vi "genIOLInsertion.vi"(11 "Arm ID Ind":i32) -> (0 "zVisTraj":dbl[](array[numeric]) format="%_6g", 1 "yVisTraj":dbl[](array[numeric]) format="%_6g", 2 "xVisTraj":dbl[](array[numeric]) format="%_6g")   [LabVIEW 2016]
uses:
  <vilib>/Analysis/NI_AALBase.lvlib
  <vilib>/Analysis/1siggen.llb/Ramp Pattern by Samples.vi
  <vilib>/gmath/NI_Gmath.lvlib
panel:
  in  "Total Time":dbl=60.0
  in  "Tip out Posit":dbl[](array[numeric])=[0.0, 0.0, 0.0] caption="Position [mm]" format="%#.3f"
  in  "Cycle Time [sec]":dbl[](array[numeric])=[60.0, 90.0, 120.0]
  in  "Sampling Rate [Hz]":i32=1000
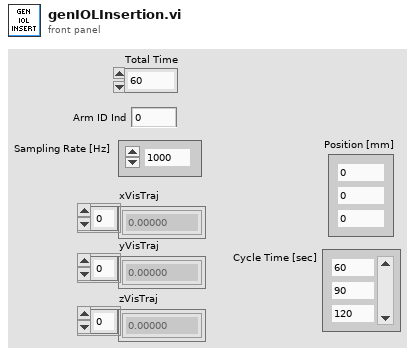
[diagram p1: front panel]
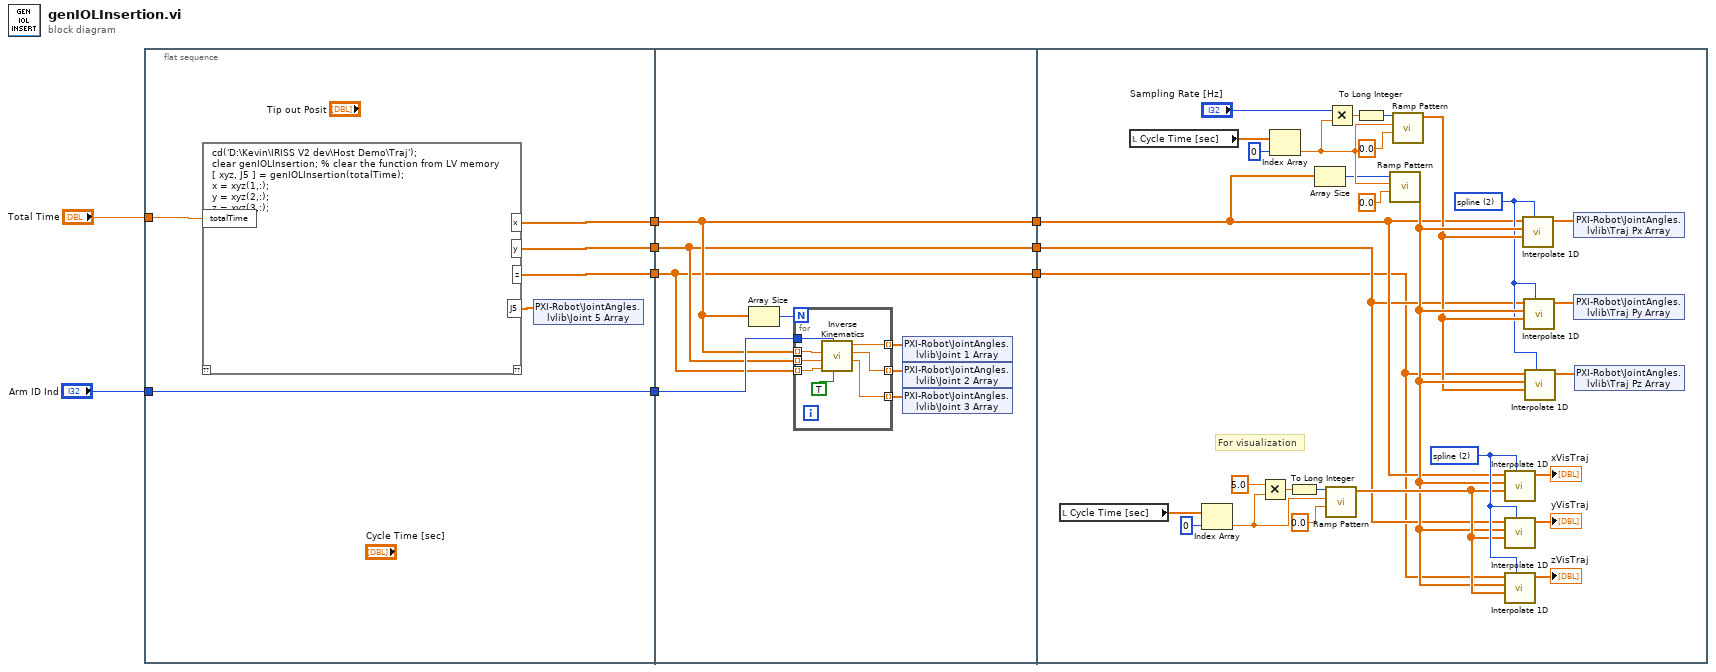
[diagram p0: block diagram]
diagram:
  n1 = flat-sequence {
    tunnel: "Arm ID Ind" -> [w14]
    tunnel: [w14] -> w8
    tunnel: [w13] -> w4
    tunnel: [w12] -> w3
    tunnel: [w11] -> w2
    tunnel: "Total Time" -> [w10]
    tunnel: w8 -> [w23]
    tunnel: [w18] -> w7
    tunnel: [w17] -> w6
    tunnel: [w16] -> w5
    tunnel: w4 -> [w18]
    tunnel: w3 -> [w17]
    tunnel: w2 -> [w16]
    tunnel: w7 -> [w34]
    tunnel: w6 -> [w33]
    tunnel: w5 -> [w32]
    frame #0 {
      n2 = script code="cd('D:\\Kevin\\IRISS V2 dev\\Host Demo\\Traj');\nclear genIOLInsertion; % clear the function from LV memory\n[ xyz, J5 ] = genIOLInsertion(totalTime);\nx = xyz(1,:);\ny = xyz(2,:);\nz = xyz(3,:);"("totalTime"=w10) -> ("x"=w13:dbl[], "y"=w12:dbl[], "z"=w11:dbl[], "J5"=w15:dbl[])  [unwired: 1 in, 1 out]
      n3 = shared-variable "PXI-Robot\\JointAngles.lvlib\\Joint 5 Array"(w15) -> ()  [unwired: 1 in, 1 out]
    }
    frame #1 {
      n4 = Array Size(array=w18) -> (size(s)=w22:i32)
      n5 = for {
        N: w22 -> [_]
        tunnel: w23 -> [w27]
        tunnel: w18 -> [w31] mode=indexing
        tunnel: w17 -> [w30] mode=indexing
        tunnel: w16 -> [w29] mode=indexing
        tunnel: [w26] -> w21 mode=indexing
        tunnel: [w25] -> w20 mode=indexing
        tunnel: [w24] -> w19 mode=indexing
        n6 = call "Inverse Kinematics.vi"(6:TRUE ("isToolTipInsideEye"), "armID"=w27, "z"=w29, "y"=w30, "x"=w31) -> ("j3"=w24:dbl, "j2"=w25:dbl, "j1"=w26:dbl)  [unwired: 3 in, 1 out]
      }
      n7 = shared-variable "PXI-Robot\\JointAngles.lvlib\\Joint 1 Array"(w21) -> ()  [unwired: 1 in, 1 out]
      n8 = shared-variable "PXI-Robot\\JointAngles.lvlib\\Joint 2 Array"(w20) -> ()  [unwired: 1 in, 1 out]
      n9 = shared-variable "PXI-Robot\\JointAngles.lvlib\\Joint 3 Array"(w19) -> ()  [unwired: 1 in, 1 out]
    }
    frame #2 {
      w49 = 2 items=["nearest", "linear", "spline", "cubic Hermite", "Lagrange"] ("method")
      w35 = 2 items=["nearest", "linear", "spline", "cubic Hermite", "Lagrange"] ("method")
      # "For visualization"
      n10 = local read "Cycle Time [sec]"() -> (w43:dbl[])
      n11 = local read "Cycle Time [sec]"() -> (w61:dbl[])
      n12 = Index Array(array=w43, index=0) -> (element=w44:dbl)
      n13 = Multiply(x=5.0, y=w44) -> (x*y=w46:dbl)
      n14 = Index Array(array=w61, index=0) -> (element=w54:dbl)
      n15 = To Long Integer(number=w46) -> (32bit integer=w47:i32)
      n16 = Array Size(array=w34) -> (size(s)=w53:i32)
      n17 = call-poly <vilib>:"Ramp Pattern.vi"("start"=0.0, "end"=w44, "samples"=w47) -> ("Ramp Pattern"=w41:dbl[])  [unwired: 7 in, 1 out]
      n18 = Multiply(x="Sampling Rate [Hz]", y=w54) -> (x*y=w57:dbl)
      n19 = To Long Integer(number=w57) -> (32bit integer=w58:i32)
      n20 = call-poly <vilib>:"Ramp Pattern.vi"("start"=0.0, "end"=w54, "samples"=w53) -> ("Ramp Pattern"=w37:dbl[])  [unwired: 7 in, 1 out]
      n21 = call-poly <vilib>:"Ramp Pattern.vi"("start"=0.0, "end"=w54, "samples"=w58) -> ("Ramp Pattern"=w36:dbl[])  [unwired: 7 in, 1 out]
      n22 = call <vilib>:"Interpolate 1D.vi"("method"=w49, "xi"=w41, "X"=w37, "Y"=w34) -> ("yi"=→"xVisTraj":dbl[])  [unwired: 5 in, 2 out]
      n23 = call <vilib>:"Interpolate 1D.vi"("method"=w49, "xi"=w41, "X"=w37, "Y"=w33) -> ("yi"=→"yVisTraj":dbl[])  [unwired: 5 in, 2 out]
      n24 = call <vilib>:"Interpolate 1D.vi"("method"=w49, "xi"=w41, "X"=w37, "Y"=w32) -> ("yi"=→"zVisTraj":dbl[])  [unwired: 5 in, 2 out]
      n25 = call <vilib>:"Interpolate 1D.vi"("method"=w35, "xi"=w36, "X"=w37, "Y"=w34) -> ("yi"=w51:dbl[])  [unwired: 5 in, 2 out]
      n26 = call <vilib>:"Interpolate 1D.vi"("method"=w35, "xi"=w36, "X"=w37, "Y"=w33) -> ("yi"=w52:dbl[])  [unwired: 5 in, 2 out]
      n27 = call <vilib>:"Interpolate 1D.vi"("method"=w35, "xi"=w36, "X"=w37, "Y"=w32) -> ("yi"=w50:dbl[])  [unwired: 5 in, 2 out]
      n28 = shared-variable "PXI-Robot\\JointAngles.lvlib\\Traj Px Array"(w51) -> ()  [unwired: 1 in, 1 out]
      n29 = shared-variable "PXI-Robot\\JointAngles.lvlib\\Traj Py Array"(w52) -> ()  [unwired: 1 in, 1 out]
      n30 = shared-variable "PXI-Robot\\JointAngles.lvlib\\Traj Pz Array"(w50) -> ()  [unwired: 1 in, 1 out]
    }
  }
